vi "checkCRC.vi"(8 "error in (no error)":errorcluster, 10 "CRC":u16, 11 "FrameParser in":refnum<class "FrameParser.lvclass">) -> (0 "error out":errorcluster, 2 "Valid?":bool, 3 "FrameParser out":refnum<class "FrameParser.lvclass">)   [LabVIEW 2015, in "RTModbus.lvlib" / "FrameParser.lvclass"]
uses:
  FrameParser.lvclass
  FrameParser.lvclass/FrameParser.ctl
  CRC/CRC.lvclass
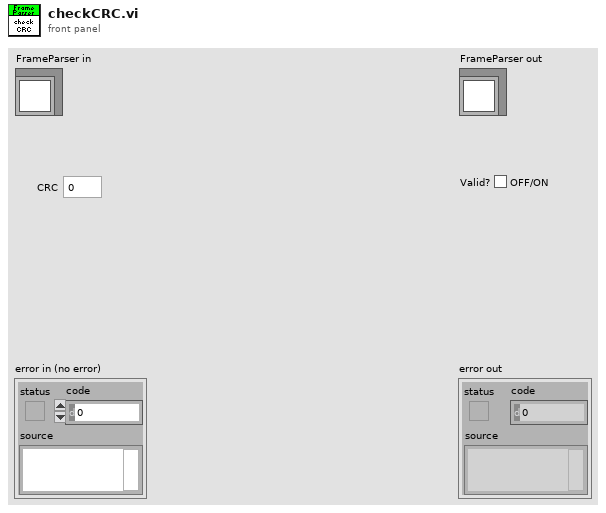
[diagram p1: front panel]
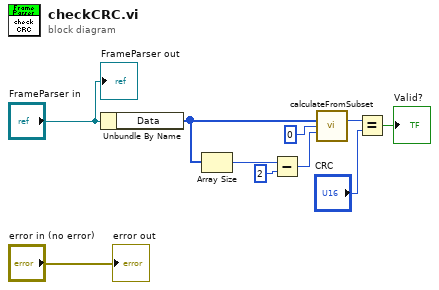
[diagram p0: block diagram]
diagram:
  n1 = Unbundle By Name("FrameParser in") -> ("Data"=w9:u8[])
  n2 = Array Size(array=w9) -> (size(s)=w8:i32)
  n3 = Subtract(x=w8, y=2) -> (x-y=w6:i32)
  n4 = call "calculateFromSubset.vi"("Data"=w9, "StartIndex"=0, "Length"=w6) -> ("CRC"=w4:u16)  [unwired: 10 in, 2 out]
  n5 = Equal?(x=w4, y="CRC") -> (x = y?=→"Valid?":bool)
  "error out" <- "error in (no error)"
  "FrameParser out" <- "FrameParser in"
